vi "Create Sessions - 1Sess.vi"(7 "serial configuration":T1, 8 "error in":errorcluster, 9 "reset":bool, 11 "session reservation in":refnum<class "Session Reservation.lvclass">) -> (0 "error out":errorcluster, 1 "channel list":string, 2 "session":refnum<visa-resource-name>, 3 "session reservation out":refnum<class "Session Reservation.lvclass">)   [LabVIEW 2020, in "MeasurementLink 34401.lvlib"]
doc: "Create the 34401 driver session from the <b>session reservation in</b>. Returns an error if more than one 34401 session has been reserved. Use \"Create Session - NSess.vi\" for multiple sessions."
uses:
  MeasurementLink 34401.lvlib
  <vilib>/MeasurementLink/MeasurementLink Session Management/Session Reservation/Session Reservation.lvclass
  7f77feb2-d2b5-4acd-8f0f-f1b24b7d1641.vi
  Instrument/Instrument.lvclass
  C:/Program Files/National Instruments/LabVIEW 2020/vi.lib/MeasurementLink/MeasurementLink Instrument/IInstrument/IInstrument.lvclass
  <vilib>/MeasurementLink/MeasurementLink Session Management/Session Reservation/Create Sessions Dispatcher.vi
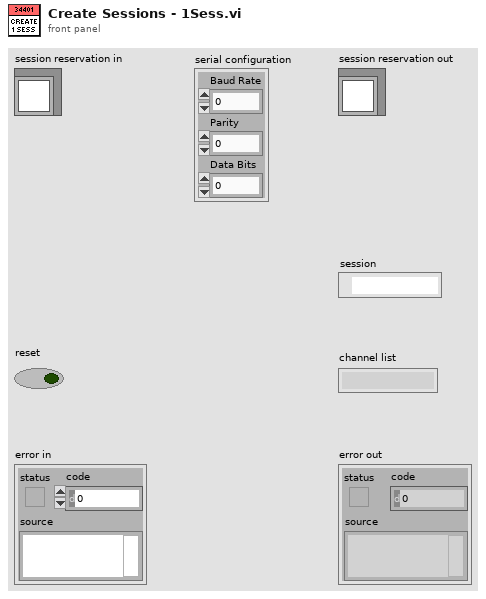
[diagram p1: front panel]
types:
  T1 = cluster{"Baud Rate":u32, "Parity":u16, "Data Bits":u16}
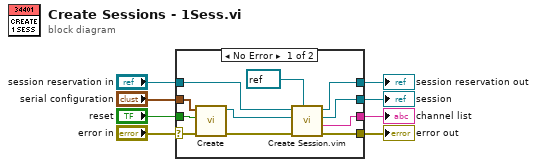
[diagram p0: block diagram]
diagram:
  n1 = case shown="No Error" "error in" {
    selector: "error in" -> [w18 w21]
    tunnel: [w16 w21] -> w7
    tunnel: [w19 w20] -> w5
    tunnel: "session reservation in" -> [w12 w20]
    tunnel: "reset" -> [w17 _]
    tunnel: [w15 _] -> w3
    tunnel: [w14 _] -> w1
    tunnel: "serial configuration" -> [w10 _]
    frame No Error {
      n2 = call "Create.vi"("error in"=w18, "reset"=w17, "serial configuration"=w10) -> ("error out"=w11:errorcluster, "instrument out"=w13:refnum<class "Instrument.lvclass">)  [unwired: 7 in]
      n3 = call "Create Session.vim"("session type"=refnum<visa-resource-name> refnum ("session"), "error in"=w11, "instrument"=w13, "session reservation in"=w12) -> ("error out"=w16:errorcluster, "channel list"=w15:string, "session"=w14:refnum<visa-resource-name>, "session reservation out"=w19:refnum<class "Session Reservation.lvclass">)  [unwired: 4 in]
    }
    frame Error {
    }
  }
  "error out" <- w7
  "session reservation out" <- w5
  "channel list" <- w3
  "session" <- w1
